vi "Read Anything.vi"(7 "Type of Anything":variant, 8 "Error In":errorcluster, 9 "Section Name (Name of \"Type of Anything\")":string, 11 "Path (dialog)":path) -> (0 "Error Out":errorcluster, 1 "Found?":bool, 3 "Anything":variant)   [LabVIEW 2020]
doc: "This VI is designed to read data from a file written by <B>Write Anything.vi</B>. If the data type definition has changed since it was written to file, this VI will still read and fill out any elements of the cluster that have the same name. Any elements for which it cannot find a name match in the file will be supplied with their datatype's default value.\n\nFreeware from Moore Good Ideas, www.mooregoodideas.com. Do not remove this line."
uses:
  Koop/KObject Class/KObject.lvclass
  <vilib>/Utility/VariantDataType/VariantType.lvlib
  <vilib>/Utility/Data Type/NI_Data Type.lvlib
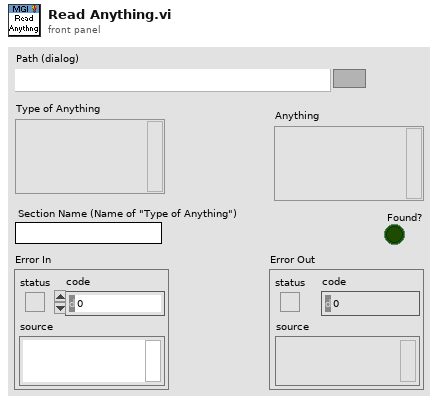
[diagram p1: front panel]
types:
  T1 = typedef "VariantType.lvlib/Type.ctl" = enum8{"Invalid Type", "Void", "I8", "I16", "I32", "I64", "U8", "U16", "U32", "U64", "Single Float", "Double Float", "Extended Float", "Single Complex", "Double Complex", "Extended Complex", "Enum U8", "Enum U16", "Enum U32", "Enum U64", "Single Float With Unit", "Double Float With Unit", "Extended Float With Unit", "Single Complex with Unit", "Double Complex with Unit", "Extended Complex with Unit", "Boolean", "String", "Path", "Picture", "Tag", "Array", "Cluster", "Variant", "LV Variant", "Waveform", "Timestamp", "Digital Waveform", "Digital Data", "ExpressData", "Refnum", "External Data", "VI", "Poly VI", "LabVIEW Class Instance", "Fixed Point"}
  T2 = typedef "NI_Data Type.lvlib/Data Type.ctl" = enum8{"Invalid Type", "Void", "I8", "I16", "I32", "I64", "U8", "U16", "U32", "U64", "Single Float", "Double Float", "Extended Float", "Single Complex", "Double Complex", "Extended Complex", "Enum U8", "Enum U16", "Enum U32", "Enum U64", "Single Float With Unit", "Double Float With Unit", "Extended Float With Unit", "Single Complex with Unit", "Double Complex with Unit", "Extended Complex with Unit", "Boolean", "String", "Path", "Picture", "Tag", "Array", "Cluster", "Variant", "LV Variant", "Waveform", "Timestamp", "Digital Waveform", "Digital Data", "ExpressData", "Refnum", "External Data", "VI", "Poly VI", "LabVIEW Class Instance", "Fixed Point", "Set Collection", "Map Collection"}
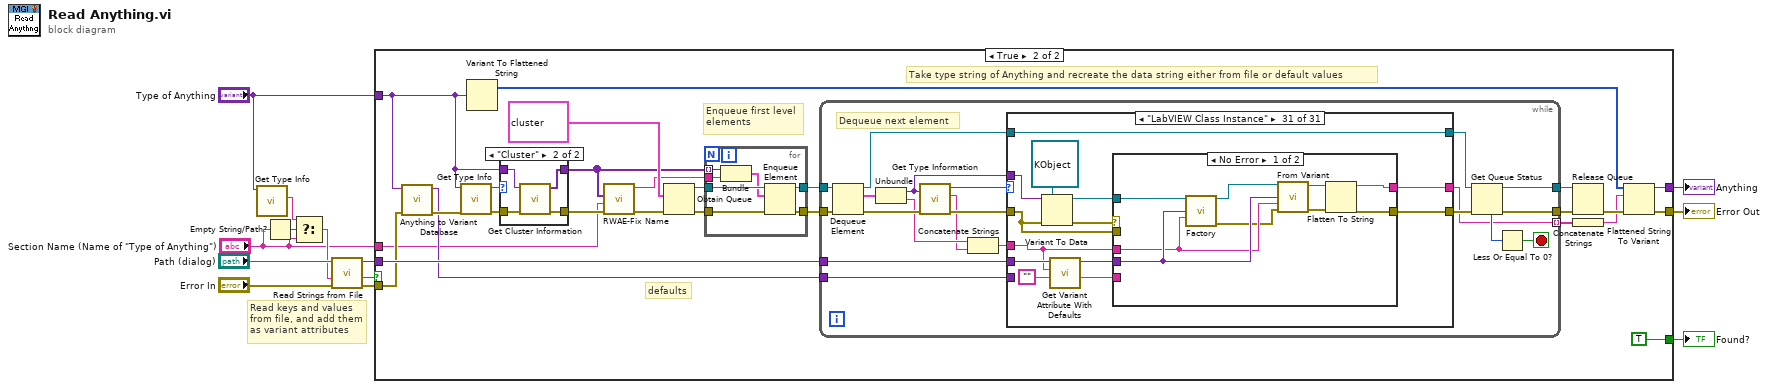
[diagram p0: block diagram]
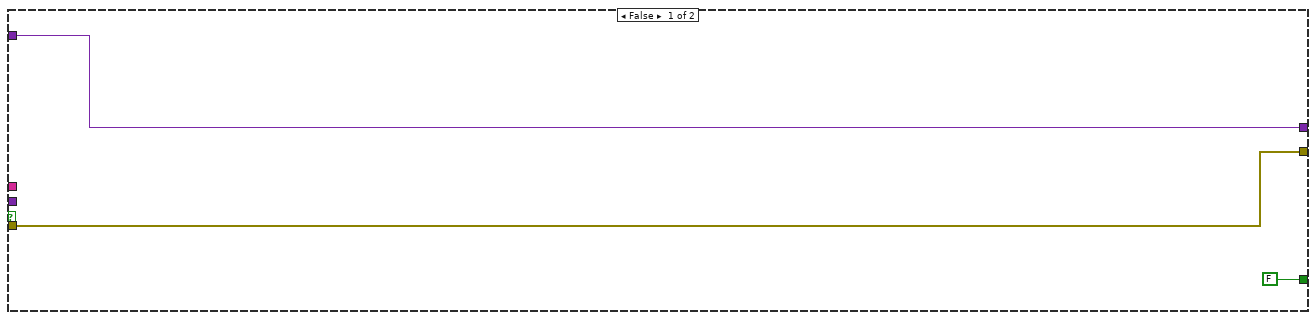
[diagram p2: hidden frame]
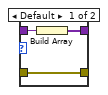
[diagram p3: hidden frame]
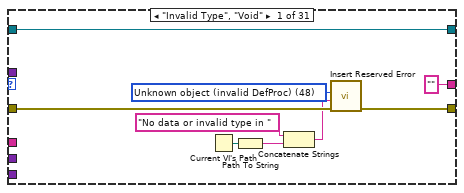
[diagram p4: hidden frame]
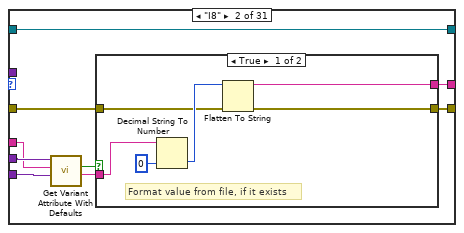
[diagram p5: hidden frame]
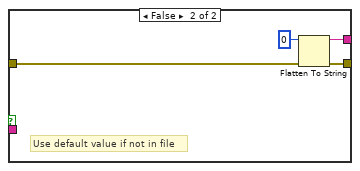
[diagram p6: hidden frame]
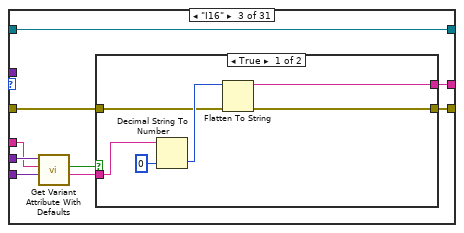
[diagram p7: hidden frame]
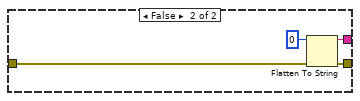
[diagram p8: hidden frame]
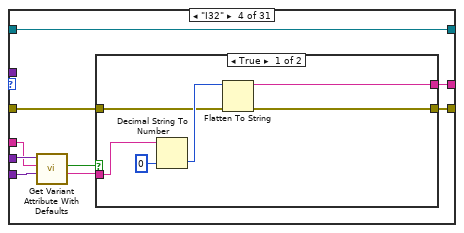
[diagram p9: hidden frame]
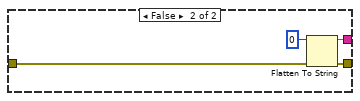
[diagram p10: hidden frame]
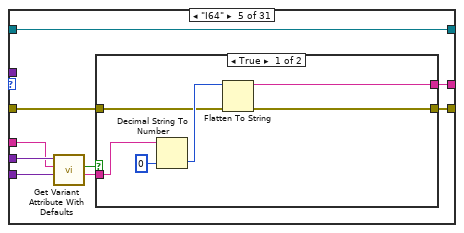
[diagram p11: hidden frame]
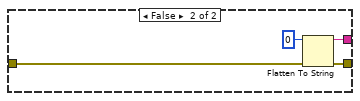
[diagram p12: hidden frame]
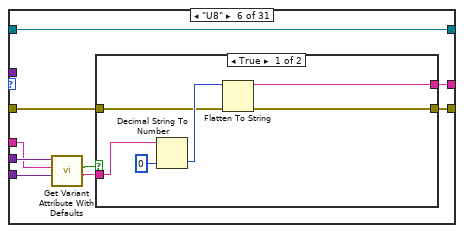
[diagram p13: hidden frame]
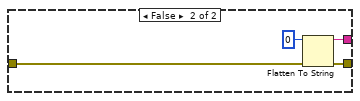
[diagram p14: hidden frame]
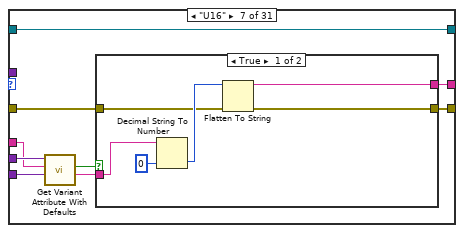
[diagram p15: hidden frame]
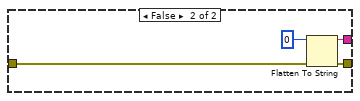
[diagram p16: hidden frame]
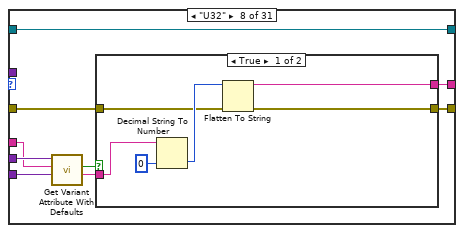
[diagram p17: hidden frame]
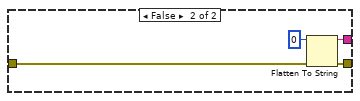
[diagram p18: hidden frame]
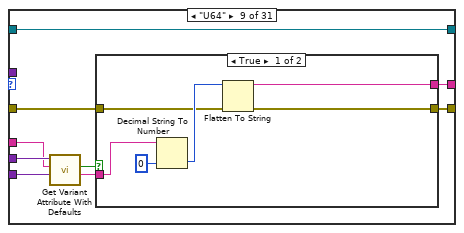
[diagram p19: hidden frame]
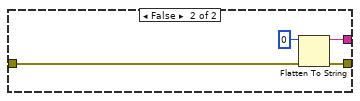
[diagram p20: hidden frame]
diagram:
  # "Read keys and values from file, and add them as variant attributes"
  n1 = call "Get Type Info.vi"("Variant"="Type of Anything") -> ("Name"=w3:string)  [unwired: 8 in, 2 out]
  n2 = Empty String/Path?(string/path="Section Name (Name of \"Type of Anything\")") -> (empty?=w5:bool)
  n3 = Select(t=w3, s=w5, f="Section Name (Name of \"Type of Anything\")") -> (s? t:f=w4:string)
  n4 = call "Read Strings from File.vi"("Error In"="Error In", "Section Name"=w4, "Path"="Path (dialog)") -> ("Error Out"=w11:errorcluster, "Found?"=w8:bool, "Variant Database"=w7:variant)  [unwired: 6 in]
  n5 = case shown="True" w8 {
    tunnel: [w15 w41] -> w13
    tunnel: [w16 w40] -> w12
    tunnel: "Type of Anything" -> [w16 w23]
    tunnel: w11 -> [w15 w25]
    tunnel: [FALSE TRUE] -> w9
    tunnel: w7 -> [_ w28]
    tunnel: "Section Name (Name of \"Type of Anything\")" -> [_ w18]
    frame False {
    }
    frame True {
      # "defaults"
      # "Enqueue first level\nelements"
      # "Take type string of Anything and recreate the data string either from file or default values"
      n6 = call "Anything to Variant Database.vi"("Error In"=w25, "Type of Anything"=w23) -> ("Error Out"=w24:errorcluster, "Variant Database"=w22:variant)  [unwired: 8 in]
      n7 = call "Get Type Info.vi"("Error In"=w24, "Variant"=w23) -> ("Error Out"=w26:errorcluster, "Type Enum"=w27:T1)  [unwired: 7 in, 1 out]
      n8 = Variant To Flattened String(Variant=w23) -> (1:w42:i16[])  [unwired: 1 out]
      n9 = case shown="\"Cluster\"" w27 {
        tunnel: [w45 w48] -> w21
        tunnel: w26 -> [w45 w49]
        tunnel: w23 -> [w44 w47]
        tunnel: [w43 w46] -> w19
        frame Default {
          n10 = Build Array(w44) -> (w43:variant[])
        }
        frame "Cluster" {
          n11 = call <vilib>:"Get Cluster Information.vi"("error in (no error)"=w49, "variant"=w47) -> ("error out"=w48:errorcluster, "cluster elements"=w46:variant[])  [unwired: 8 in]
        }
      }
      n12 = call "RWAE-Fix Name.vi"("error in (no error)"=w21, "Section Name (Name of \"Anything\")"=w18, "Cluster Elements in"=w19) -> ("error out"=w20:errorcluster, "Name"=w17:string)  [unwired: 7 in]
      n13 = Obtain Queue(element data type=cluster{"Variant":variant, "Name":string} {"Variant"=variant, "Name"=""}, error in (no error)=w20) -> (queue out=w38:refnum<queue>, error out=w31:errorcluster)  [unwired: 3 in, 1 out]
      n14 = for {
        tunnel: w38 -> [w56]
        tunnel: [w55] -> w37
        tunnel: [w54] -> w36
        tunnel: w19 -> [w53] mode=indexing
        tunnel: w17 -> [w52]
        tunnel: w31 -> [w51]
        n15 = Bundle("Variant"=w53, "Name"=w52) -> (w50:cluster{"Variant":variant, "Name":string})  [unwired: 1 in]
        n16 = Enqueue Element(queue=w56, element=w50, error in (no error)=w51) -> (queue out=w54:refnum<queue>, error out=w55:errorcluster)  [unwired: 1 in, 1 out]
      }
      n17 = while {
        tunnel: w37 -> [w75]
        tunnel: [w70] -> w35
        tunnel: w28 -> [w62]
        tunnel: [w59] -> w39 mode=indexing
        tunnel: w36 -> [w72]
        tunnel: [w66] -> w33
        tunnel: w22 -> [w58]
        stop <- w67 stop-if-true
        # "Dequeue next element"
        n18 = Dequeue Element(queue=w72, error in (no error)=w75) -> (queue out=w73:refnum<queue>, element=w65:cluster{"Variant":variant, "Name":string}, error out=w74:errorcluster)  [unwired: 1 in, 1 out]
        n19 = Unbundle(w65) -> ("Variant"=w61:variant, "Name"=w63:string)
        n20 = call <vilib>:"Get Type Information.vi"("error in (no error)"=w74, "variant"=w61) -> ("error out"=w76:errorcluster, "name"=w60:string, "type"=w57:T2)  [unwired: 5 in, 2 out]
        n21 = Concatenate Strings(w63, w60) -> (w64:string)
        n22 = case shown="\"LabVIEW Class Instance\"" w57 {
          tunnel: [w79 w94 w113 w132 w151 w170 w189 w208 w227 w246 w265 w284 w303 w322 w341 w361 w387 w413 w439 w464 w483 w500 w517 w539 w568 w597 w626 w655 w683 w695 w719] -> w71
          tunnel: w76 -> [w80 w93 w112 w131 w150 w169 w188 w207 w226 w245 w264 w283 w302 w321 w340 w360 w386 w412 w438 w463 w482 w499 w523 w538 w567 w596 w625 w654 w684 w694 w718]
          tunnel: w64 -> [_ w87 w106 w125 w144 w163 w182 w201 w222 w241 w259 w279 w297 w317 w336 w354 w380 w407 w433 w457 w478 w494 w512 w534 w563 w591 w619 w649 w679 w687 w716]
          tunnel: ["" ("data string") w92 w111 w130 w149 w168 w187 w206 w225 w244 w263 w282 w301 w320 w339 w359 w385 w411 w437 w462 w481 w498 "" w537 w566 w595 w624 w653 w681 w693 w720] -> w59
          tunnel: w61 -> [_ _ _ _ _ _ _ _ _ _ _ _ _ _ _ w358 w384 w410 w436 _ _ _ w522 _ _ _ _ _ w682 _ w721]
          tunnel: w73 -> [w81 w91 w110 w129 w148 w167 w186 w205 w224 w243 w262 w281 w300 w319 w338 w357 w383 w409 w435 w461 w480 w497 w518 w536 w565 w594 w623 w652 w686 w692 w728]
          tunnel: [w81 w91 w110 w129 w148 w167 w186 w205 w224 w243 w262 w281 w300 w319 w338 w357 w383 w409 w435 w461 w480 w497 w516 w536 w565 w594 w623 w652 w685 w692 w728] -> w69
          tunnel: w62 -> [_ w88 w107 w126 w145 w164 w183 w202 w223 w242 w260 w280 w298 w318 w337 w356 w381 w408 w434 w458 w479 w495 _ w535 w564 w593 w622 w650 w680 w690 w726]
          tunnel: w58 -> [_ w86 w105 w124 w143 w162 w181 w200 w219 w238 w257 w276 w295 w314 w333 w352 w378 w404 w430 w456 w475 w492 _ w531 w560 w589 w618 w647 w677 _ _]
          frame "Invalid Type", "Void" {
            w77 = u16 48 items=["No error", "Argument error", "Memory is full", "Out of zone", "End of file", "File already open", "Generic file I/O error", "File not found", "File permission error", "Disk is full", "Duplicate path", "Too many files open", "System feature not enabled", "Resource file not found", "Cannot add resource", "Resource not found", "Image not found", "Image memory error", "Pen does not exist", "Config type invalid", "Config token not found", "Config parse error", "Config memory error", "Bad external code format", "Bad external code offset", "External code not present", "Null window", "Destroy window error", "Null menu", "Print aborted", "Bad print record", "Print driver error", "Windows error during printing", "Memory error during printing", "Print dialog error", "Generic print error", "Invalid device refnum", "Device not found", "Device parameter error", "Device unit error", "Cannot open device", "Device call aborted", "Generic error", "Cancelled by user", "Object ID too low", "Object ID too high", "Object not in heap", "Unknown heap", "Unknown object (invalid DefProc)", "Unknown object (DefProc not in table)", "Message out of range", "Invalid (null) method", "Unknown message", "Manager call not supported", "Bad address", "Network operation in progress", "Network operation timed out", "Connection is busy", "Network attribute not supported", "Network error", "Address in use", "System out of memory", "Connection aborted", "Connection refused", "Not connected", "Already connected", "Connection closed", "Initialization error (interapplication manager)", "Bad occurrence", "Wait on unbound occurrence handler", "Occurrence queue overflow", "Datalog type conflict", "Unused", "Unrecognized type (interapplication manager)", "Memory corrupt", "Failed to make temporary DLL", "Old CIN version", "Drag socket not found", "Failed to load drop-object", "Failed to register OLE object", "Failed to release OLE object", "Format specifier type mismatch", "Unknown format specifier", "Too few format specifiers", "Too many format specifiers", "Scan failed", "Newer CIN version", "OLE Convert", "Runtime menu error", "Password tampered", "Unknown error code"] ("Reserved Error Code")
            n23 = Current VI's Path() -> (path=w83:path)
            n24 = Path To String(path=w83) -> (string=w82:string)
            n25 = Concatenate Strings("No data or invalid type in " ("string"), w82) -> (w78:string)
            n26 = call "Insert Reserved Error.vi"("error in (no error)"=w80, "non-standard source (\"\")"=w78, "Reserved Error Code"=w77) -> ("error out"=w79:errorcluster)  [unwired: 4 in]
          }
          frame "I8" {
            n27 = call "Get Variant Attribute With Defaults.vi"("Variant Database defaults"=w86, "name"=w87, "Variant Database from file"=w88) -> ("values"=w89:string, "found"=w90:bool)  [unwired: 6 in, 1 out]
            n28 = case shown="True" w90 {
              tunnel: w89 -> [w95 _]
              tunnel: [w98 w101] -> w94
              tunnel: w93 -> [w97 w102]
              tunnel: [w99 w104] -> w92
              frame True {
                # "Format value from file, if it exists"
                n29 = Decimal String To Number(string=w95, default (0L)=i8 0 ("default (0 I32)")) -> (number=w100:i8)  [unwired: 1 in, 1 out]
                n30 = Flatten To String(anything=w100, error in (no error)=w97) -> (data string=w99:string, error out=w98:errorcluster)  [unwired: 2 in, 1 out]
              }
              frame False {
                # "Use default value if not in file"
                n31 = Flatten To String(anything=i8 0, error in (no error)=w102) -> (data string=w104:string, error out=w101:errorcluster)  [unwired: 2 in, 1 out]
              }
            }
          }
          frame "I16" {
            n32 = call "Get Variant Attribute With Defaults.vi"("Variant Database defaults"=w105, "name"=w106, "Variant Database from file"=w107) -> ("values"=w108:string, "found"=w109:bool)  [unwired: 6 in, 1 out]
            n33 = case shown="True" w109 {
              tunnel: w108 -> [w114 _]
              tunnel: [w117 w120] -> w113
              tunnel: w112 -> [w116 w121]
              tunnel: [w118 w123] -> w111
              frame True {
                n34 = Decimal String To Number(string=w114, default (0L)=i16 0 ("default (0 I32)")) -> (number=w119:i16)  [unwired: 1 in, 1 out]
                n35 = Flatten To String(anything=w119, error in (no error)=w116) -> (data string=w118:string, error out=w117:errorcluster)  [unwired: 2 in, 1 out]
              }
              frame False {
                n36 = Flatten To String(anything=i16 0, error in (no error)=w121) -> (data string=w123:string, error out=w120:errorcluster)  [unwired: 2 in, 1 out]
              }
            }
          }
          frame "I32" {
            n37 = call "Get Variant Attribute With Defaults.vi"("Variant Database defaults"=w124, "name"=w125, "Variant Database from file"=w126) -> ("values"=w127:string, "found"=w128:bool)  [unwired: 6 in, 1 out]
            n38 = case shown="True" w128 {
              tunnel: w127 -> [w133 _]
              tunnel: [w136 w139] -> w132
              tunnel: w131 -> [w135 w140]
              tunnel: [w137 w142] -> w130
              frame True {
                n39 = Decimal String To Number(string=w133, default (0L)=0 ("default (0 I32)")) -> (number=w138:i32)  [unwired: 1 in, 1 out]
                n40 = Flatten To String(anything=w138, error in (no error)=w135) -> (data string=w137:string, error out=w136:errorcluster)  [unwired: 2 in, 1 out]
              }
              frame False {
                n41 = Flatten To String(anything=0, error in (no error)=w140) -> (data string=w142:string, error out=w139:errorcluster)  [unwired: 2 in, 1 out]
              }
            }
          }
          frame "I64" {
            n42 = call "Get Variant Attribute With Defaults.vi"("Variant Database defaults"=w143, "name"=w144, "Variant Database from file"=w145) -> ("values"=w146:string, "found"=w147:bool)  [unwired: 6 in, 1 out]
            n43 = case shown="True" w147 {
              tunnel: w146 -> [w152 _]
              tunnel: [w155 w158] -> w151
              tunnel: w150 -> [w154 w159]
              tunnel: [w156 w161] -> w149
              frame True {
                n44 = Decimal String To Number(string=w152, default (0L)=i64 0 ("default (0 I32)")) -> (number=w157:i64)  [unwired: 1 in, 1 out]
                n45 = Flatten To String(anything=w157, error in (no error)=w154) -> (data string=w156:string, error out=w155:errorcluster)  [unwired: 2 in, 1 out]
              }
              frame False {
                n46 = Flatten To String(anything=i64 0, error in (no error)=w159) -> (data string=w161:string, error out=w158:errorcluster)  [unwired: 2 in, 1 out]
              }
            }
          }
          frame "U8" {
            n47 = call "Get Variant Attribute With Defaults.vi"("Variant Database defaults"=w162, "name"=w163, "Variant Database from file"=w164) -> ("values"=w165:string, "found"=w166:bool)  [unwired: 6 in, 1 out]
            n48 = case shown="True" w166 {
              tunnel: w165 -> [w171 _]
              tunnel: [w174 w177] -> w170
              tunnel: w169 -> [w173 w178]
              tunnel: [w175 w180] -> w168
              frame True {
                n49 = Decimal String To Number(string=w171, default (0L)=u8 0 ("default (0 I32)")) -> (number=w176:u8)  [unwired: 1 in, 1 out]
                n50 = Flatten To String(anything=w176, error in (no error)=w173) -> (data string=w175:string, error out=w174:errorcluster)  [unwired: 2 in, 1 out]
              }
              frame False {
                n51 = Flatten To String(anything=u8 0, error in (no error)=w178) -> (data string=w180:string, error out=w177:errorcluster)  [unwired: 2 in, 1 out]
              }
            }
          }
          frame "U16" {
            n52 = call "Get Variant Attribute With Defaults.vi"("Variant Database defaults"=w181, "name"=w182, "Variant Database from file"=w183) -> ("values"=w184:string, "found"=w185:bool)  [unwired: 6 in, 1 out]
            n53 = case shown="True" w185 {
              tunnel: w184 -> [w190 _]
              tunnel: [w193 w196] -> w189
              tunnel: w188 -> [w192 w197]
              tunnel: [w194 w199] -> w187
              frame True {
                n54 = Decimal String To Number(string=w190, default (0L)=u16 0 ("default (0 I32)")) -> (number=w195:u16)  [unwired: 1 in, 1 out]
                n55 = Flatten To String(anything=w195, error in (no error)=w192) -> (data string=w194:string, error out=w193:errorcluster)  [unwired: 2 in, 1 out]
              }
              frame False {
                n56 = Flatten To String(anything=u16 0, error in (no error)=w197) -> (data string=w199:string, error out=w196:errorcluster)  [unwired: 2 in, 1 out]
              }
            }
          }
          frame "U32" {
            n57 = call "Get Variant Attribute With Defaults.vi"("Variant Database defaults"=w200, "name"=w201, "Variant Database from file"=w202) -> ("values"=w203:string, "found"=w204:bool)  [unwired: 6 in, 1 out]
            n58 = case shown="True" w204 {
              tunnel: w203 -> [w209 _]
              tunnel: [w212 w215] -> w208
              tunnel: w207 -> [w211 w216]
              tunnel: [w213 w218] -> w206
              frame True {
                n59 = Decimal String To Number(string=w209, default (0L)=u32 0 ("default (0 I32)")) -> (number=w214:u32)  [unwired: 1 in, 1 out]
                n60 = Flatten To String(anything=w214, error in (no error)=w211) -> (data string=w213:string, error out=w212:errorcluster)  [unwired: 2 in, 1 out]
              }
              frame False {
                n61 = Flatten To String(anything=u32 0, error in (no error)=w216) -> (data string=w218:string, error out=w215:errorcluster)  [unwired: 2 in, 1 out]
              }
            }
          }
          frame "U64" {
            n62 = call "Get Variant Attribute With Defaults.vi"("Variant Database defaults"=w219, "name"=w222, "Variant Database from file"=w223) -> ("values"=w221:string, "found"=w220:bool)  [unwired: 6 in, 1 out]
            n63 = case shown="True" w220 {
              tunnel: w221 -> [w228 _]
              tunnel: [w231 w234] -> w227
              tunnel: w226 -> [w230 w235]
              tunnel: [w232 w237] -> w225
              frame True {
                n64 = Decimal String To Number(string=w228, default (0L)=u64 0 ("default (0 I32)")) -> (number=w233:u64)  [unwired: 1 in, 1 out]
                n65 = Flatten To String(anything=w233, error in (no error)=w230) -> (data string=w232:string, error out=w231:errorcluster)  [unwired: 2 in, 1 out]
              }
              frame False {
                n66 = Flatten To String(anything=u64 0, error in (no error)=w235) -> (data string=w237:string, error out=w234:errorcluster)  [unwired: 2 in, 1 out]
              }
            }
          }
          frame "Single Float", "Single Float With Unit" {
            n67 = call "Get Variant Attribute With Defaults.vi"("Variant Database defaults"=w238, "name"=w241, "Variant Database from file"=w242) -> ("values"=w240:string, "found"=w239:bool)  [unwired: 6 in, 1 out]
            n68 = case shown="True" w239 {
              tunnel: w240 -> [w247 _]
              tunnel: [w250 w253] -> w246
              tunnel: w245 -> [w249 w254]
              tunnel: [w251 w256] -> w244
              frame True {
                n69 = Fract/Exp String To Number(string=w247, default (0 dbl)=sgl 0.0 ("default (0 I32)")) -> (number=w252:sgl)  [unwired: 2 in, 1 out]
                n70 = Flatten To String(anything=w252, error in (no error)=w249) -> (data string=w251:string, error out=w250:errorcluster)  [unwired: 2 in, 1 out]
              }
              frame False {
                n71 = Flatten To String(anything=sgl 0.0, error in (no error)=w254) -> (data string=w256:string, error out=w253:errorcluster)  [unwired: 2 in, 1 out]
              }
            }
          }
          frame "Double Float", "Double Float With Unit" {
            n72 = call "Get Variant Attribute With Defaults.vi"("Variant Database defaults"=w257, "name"=w259, "Variant Database from file"=w260) -> ("values"=w261:string, "found"=w258:bool)  [unwired: 6 in, 1 out]
            n73 = case shown="True" w258 {
              tunnel: w261 -> [w266 _]
              tunnel: [w269 w272] -> w265
              tunnel: w264 -> [w268 w273]
              tunnel: [w270 w275] -> w263
              frame True {
                n74 = Fract/Exp String To Number(string=w266, default (0 dbl)=0.0 ("default (0 DBL)")) -> (number=w271:dbl)  [unwired: 2 in, 1 out]
                n75 = Flatten To String(anything=w271, error in (no error)=w268) -> (data string=w270:string, error out=w269:errorcluster)  [unwired: 2 in, 1 out]
              }
              frame False {
                n76 = Flatten To String(anything=0.0, error in (no error)=w273) -> (data string=w275:string, error out=w272:errorcluster)  [unwired: 2 in, 1 out]
              }
            }
          }
          frame "Extended Float", "Extended Float With Unit" {
            n77 = call "Get Variant Attribute With Defaults.vi"("Variant Database defaults"=w276, "name"=w279, "Variant Database from file"=w280) -> ("values"=w278:string, "found"=w277:bool)  [unwired: 6 in, 1 out]
            n78 = case shown="True" w277 {
              tunnel: w278 -> [w285 _]
              tunnel: [w288 w291] -> w284
              tunnel: w283 -> [w287 w292]
              tunnel: [w289 w294] -> w282
              frame True {
                n79 = Fract/Exp String To Number(string=w285, default (0 dbl)=ext 0.0 ("default (0 DBL)")) -> (number=w290:ext)  [unwired: 2 in, 1 out]
                n80 = Flatten To String(anything=w290, error in (no error)=w287) -> (data string=w289:string, error out=w288:errorcluster)  [unwired: 2 in, 1 out]
              }
              frame False {
                n81 = Flatten To String(anything=ext 0.0, error in (no error)=w292) -> (data string=w294:string, error out=w291:errorcluster)  [unwired: 2 in, 1 out]
              }
            }
          }
          frame "Single Complex", "Single Complex with Unit" {
            n82 = call "Get Variant Attribute With Defaults.vi"("Variant Database defaults"=w295, "name"=w297, "Variant Database from file"=w298) -> ("values"=w299:string, "found"=w296:bool)  [unwired: 6 in, 1 out]
            n83 = case shown="True" w296 {
              tunnel: w299 -> [w304 _]
              tunnel: [w308 w310] -> w303
              tunnel: w302 -> [w307 w311]
              tunnel: [w309 w313] -> w301
              frame True {
                n84 = Scan From String(input string=w304, default 1=csg 0.0+0.0i ("default (0 DBL)")) -> (output 1=w305:csg)  [unwired: 3 in, 3 out]
                n85 = Flatten To String(anything=w305, error in (no error)=w307) -> (data string=w309:string, error out=w308:errorcluster)  [unwired: 2 in, 1 out]
              }
              frame False {
                n86 = Flatten To String(anything=csg 0.0+0.0i, error in (no error)=w311) -> (data string=w313:string, error out=w310:errorcluster)  [unwired: 2 in, 1 out]
              }
            }
          }
          frame "Double Complex", "Double Complex with Unit" {
            n87 = call "Get Variant Attribute With Defaults.vi"("Variant Database defaults"=w314, "name"=w317, "Variant Database from file"=w318) -> ("values"=w316:string, "found"=w315:bool)  [unwired: 6 in, 1 out]
            n88 = case shown="True" w315 {
              tunnel: w316 -> [w323 _]
              tunnel: [w327 w329] -> w322
              tunnel: w321 -> [w326 w330]
              tunnel: [w328 w332] -> w320
              frame True {
                n89 = Scan From String(input string=w323, default 1=cdb 0.0+0.0i ("default (0 DBL)")) -> (output 1=w325:cdb)  [unwired: 3 in, 3 out]
                n90 = Flatten To String(anything=w325, error in (no error)=w326) -> (data string=w328:string, error out=w327:errorcluster)  [unwired: 2 in, 1 out]
              }
              frame False {
                n91 = Flatten To String(anything=cdb 0.0+0.0i, error in (no error)=w330) -> (data string=w332:string, error out=w329:errorcluster)  [unwired: 2 in, 1 out]
              }
            }
          }
          frame "Extended Complex", "Extended Complex with Unit" {
            n92 = call "Get Variant Attribute With Defaults.vi"("Variant Database defaults"=w333, "name"=w336, "Variant Database from file"=w337) -> ("values"=w335:string, "found"=w334:bool)  [unwired: 6 in, 1 out]
            n93 = case shown="True" w334 {
              tunnel: w335 -> [w342 _]
              tunnel: [w346 w348] -> w341
              tunnel: w340 -> [w345 w349]
              tunnel: [w347 w351] -> w339
              frame True {
                n94 = Scan From String(input string=w342, default 1=cxt 0.0+0.0i ("default (0 DBL)")) -> (output 1=w343:cxt)  [unwired: 3 in, 3 out]
                n95 = Flatten To String(anything=w343, error in (no error)=w345) -> (data string=w347:string, error out=w346:errorcluster)  [unwired: 2 in, 1 out]
              }
              frame False {
                n96 = Flatten To String(anything=cxt 0.0+0.0i, error in (no error)=w349) -> (data string=w351:string, error out=w348:errorcluster)  [unwired: 2 in, 1 out]
              }
            }
          }
          frame "Enum U8" {
            n97 = call "Get Variant Attribute With Defaults.vi"("Variant Database defaults"=w352, "name"=w354, "Variant Database from file"=w356) -> ("values"=w355:string, "found"=w353:bool)  [unwired: 6 in, 1 out]
            n98 = case shown="True" w353 {
              tunnel: w355 -> [w362 _]
              tunnel: [w372 w375] -> w361
              tunnel: w360 -> [w371 w376]
              tunnel: [w373 w377] -> w359
              tunnel: w358 -> [w370 _]
              frame True {
                n99 = call <vilib>:"GetNumericInfo.vi"("error in (no error)"=w371, "Variant"=w370) -> ("error out"=w363:errorcluster, "EnumNames"=w369:string[])  [unwired: 6 in, 2 out]
                n100 = Search 1D Array(1D array=w369, element=w362) -> (index of element=w368:i32)  [unwired: 1 in]
                n101 = In Range and Coerce(upper limit=255, x=w368, lower limit=0) -> (coerced(x)=w366:i32)  [unwired: 1 out]
                n102 = To Unsigned Byte Integer(number=w366) -> (unsigned 8bit integer=w367:u8)
                n103 = Flatten To String(anything=w367, error in (no error)=w363) -> (data string=w373:string, error out=w372:errorcluster)  [unwired: 2 in, 1 out]
              }
              frame False {
                n104 = Flatten To String(anything=u8 0, error in (no error)=w376) -> (data string=w377:string, error out=w375:errorcluster)  [unwired: 2 in, 1 out]
              }
            }
          }
          frame "Enum U16" {
            n105 = call "Get Variant Attribute With Defaults.vi"("Variant Database defaults"=w378, "name"=w380, "Variant Database from file"=w381) -> ("values"=w382:string, "found"=w379:bool)  [unwired: 6 in, 1 out]
            n106 = case shown="True" w379 {
              tunnel: w382 -> [w388 _]
              tunnel: [w398 w401] -> w387
              tunnel: w386 -> [w397 w402]
              tunnel: [w399 w403] -> w385
              tunnel: w384 -> [w396 _]
              frame True {
                n107 = call <vilib>:"GetNumericInfo.vi"("error in (no error)"=w397, "Variant"=w396) -> ("error out"=w389:errorcluster, "EnumNames"=w395:string[])  [unwired: 6 in, 2 out]
                n108 = Search 1D Array(1D array=w395, element=w388) -> (index of element=w394:i32)  [unwired: 1 in]
                n109 = In Range and Coerce(upper limit=u16 65535, x=w394, lower limit=0) -> (coerced(x)=w392:i32)  [unwired: 1 out]
                n110 = To Unsigned Word Integer(number=w392) -> (unsigned 16bit integer=w393:u16)
                n111 = Flatten To String(anything=w393, error in (no error)=w389) -> (data string=w399:string, error out=w398:errorcluster)  [unwired: 2 in, 1 out]
              }
              frame False {
                n112 = Flatten To String(anything=u16 0, error in (no error)=w402) -> (data string=w403:string, error out=w401:errorcluster)  [unwired: 2 in, 1 out]
              }
            }
          }
          frame "Enum U32" {
            n113 = call "Get Variant Attribute With Defaults.vi"("Variant Database defaults"=w404, "name"=w407, "Variant Database from file"=w408) -> ("values"=w406:string, "found"=w405:bool)  [unwired: 6 in, 1 out]
            n114 = case shown="True" w405 {
              tunnel: w406 -> [w414 _]
              tunnel: [w424 w427] -> w413
              tunnel: w412 -> [w423 w428]
              tunnel: [w425 w429] -> w411
              tunnel: w410 -> [w422 _]
              frame True {
                n115 = call <vilib>:"GetNumericInfo.vi"("error in (no error)"=w423, "Variant"=w422) -> ("error out"=w415:errorcluster, "EnumNames"=w421:string[])  [unwired: 6 in, 2 out]
                n116 = Search 1D Array(1D array=w421, element=w414) -> (index of element=w420:i32)  [unwired: 1 in]
                n117 = In Range and Coerce(upper limit=u32 4294967295, x=w420, lower limit=0) -> (coerced(x)=w418:u32)  [unwired: 1 out]
                n118 = To Unsigned Long Integer(number=w418) -> (unsigned 32bit integer=w419:u32)
                n119 = Flatten To String(anything=w419, error in (no error)=w415) -> (data string=w425:string, error out=w424:errorcluster)  [unwired: 2 in, 1 out]
              }
              frame False {
                n120 = Flatten To String(anything=u32 0, error in (no error)=w428) -> (data string=w429:string, error out=w427:errorcluster)  [unwired: 2 in, 1 out]
              }
            }
          }
          frame "Enum U64" {
            n121 = call "Get Variant Attribute With Defaults.vi"("Variant Database defaults"=w430, "name"=w433, "Variant Database from file"=w434) -> ("values"=w432:string, "found"=w431:bool)  [unwired: 6 in, 1 out]
            n122 = case shown="True" w431 {
              tunnel: [w450 w453] -> w439
              tunnel: w438 -> [w449 w454]
              tunnel: [w451 w455] -> w437
              tunnel: w436 -> [w448 _]
              tunnel: w432 -> [w440 _]
              frame True {
                n123 = call <vilib>:"GetNumericInfo.vi"("error in (no error)"=w449, "Variant"=w448) -> ("error out"=w441:errorcluster, "EnumNames"=w447:string[])  [unwired: 6 in, 2 out]
                n124 = Search 1D Array(1D array=w447, element=w440) -> (index of element=w446:i32)  [unwired: 1 in]
                n125 = In Range and Coerce(upper limit=u64 18446744073709551615, x=w446, lower limit=0) -> (coerced(x)=w444:u64)  [unwired: 1 out]
                n126 = To Unsigned Quad Integer(1:w444) -> (0:w445:u64)
                n127 = Flatten To String(anything=w445, error in (no error)=w441) -> (data string=w451:string, error out=w450:errorcluster)  [unwired: 2 in, 1 out]
              }
              frame False {
                n128 = Flatten To String(anything=u64 0, error in (no error)=w454) -> (data string=w455:string, error out=w453:errorcluster)  [unwired: 2 in, 1 out]
              }
            }
          }
          frame "Boolean" {
            n129 = call "Get Variant Attribute With Defaults.vi"("Variant Database defaults"=w456, "name"=w457, "Variant Database from file"=w458) -> ("values"=w459:string, "found"=w460:bool)  [unwired: 6 in, 1 out]
            n130 = case shown="True" w460 {
              tunnel: w459 -> [w465 _]
              tunnel: [w469 w472] -> w464
              tunnel: w463 -> [w466 w473]
              tunnel: [w470 w474] -> w462
              frame True {
                n131 = Equal?(x=w465, y="TRUE") -> (x = y?=w467:bool)
                n132 = Flatten To String(anything=w467, error in (no error)=w466) -> (data string=w470:string, error out=w469:errorcluster)  [unwired: 2 in, 1 out]
              }
              frame False {
                n133 = Flatten To String(anything=FALSE, error in (no error)=w473) -> (data string=w474:string, error out=w472:errorcluster)  [unwired: 2 in, 1 out]
              }
            }
          }
          frame "String" {
            n134 = call "Get Variant Attribute With Defaults.vi"("Variant Database defaults"=w475, "name"=w478, "Variant Database from file"=w479) -> ("values"=w476:string, "found"=w477:bool)  [unwired: 6 in, 1 out]
            n135 = case shown="True" w477 {
              tunnel: [w486 w489] -> w483
              tunnel: w482 -> [w485 w490]
              tunnel: [w487 w491] -> w481
              tunnel: w476 -> [w484 _]
              frame True {
                n136 = Flatten To String(anything=w484, error in (no error)=w485) -> (data string=w487:string, error out=w486:errorcluster)  [unwired: 2 in, 1 out]
              }
              frame False {
                n137 = Flatten To String(anything="", error in (no error)=w490) -> (data string=w491:string, error out=w489:errorcluster)  [unwired: 2 in, 1 out]
              }
            }
          }
          frame "Path" {
            n138 = call "Get Variant Attribute With Defaults.vi"("Variant Database defaults"=w492, "name"=w494, "Variant Database from file"=w495) -> ("values"=w493:string, "found"=w496:bool)  [unwired: 6 in, 1 out]
            n139 = case shown="True" w496 {
              tunnel: [w504 w507] -> w500
              tunnel: w499 -> [w503 w508]
              tunnel: [w505 w509] -> w498
              tunnel: w493 -> [w501 _]
              frame True {
                n140 = String To Path(string=w501) -> (path=w502:path)
                n141 = Flatten To String(anything=w502, error in (no error)=w503) -> (data string=w505:string, error out=w504:errorcluster)  [unwired: 2 in, 1 out]
              }
              frame False {
                n142 = Flatten To String(anything=path "", error in (no error)=w508) -> (data string=w509:string, error out=w507:errorcluster)  [unwired: 2 in, 1 out]
              }
            }
          }
          frame "Cluster" {
            # "Enqueue cluster elements"
            n143 = call <vilib>:"Search and Replace Pattern.vi"("string"=w512, "regular expression (\"\")"="Serialized") -> ("result string"=w511:string)  [unwired: 3 in, 1 out]
            n144 = call <vilib>:"GetClusterInfo.vi"("error in (no error)"=w523, "Variant"=w522) -> ("error out"=w519:errorcluster, "Cluster Elements"=w521:variant[])  [unwired: 8 in]
            n145 = Concatenate Strings(w511, "." ("string")) -> (w513:string)
            n146 = Reverse 1D Array(array=w521) -> (reversed array=w520:variant[])
            n147 = for {
              tunnel: w518 -> [w530]
              tunnel: w519 -> [w529]
              tunnel: [w528] -> w517
              tunnel: [w527] -> w516
              tunnel: w520 -> [w526] mode=indexing
              tunnel: w513 -> [w524]
              n148 = Bundle("ArrayElt"=w526, w524) -> (w525:cluster{"ArrayElt":variant, string})  [unwired: 1 in]
              n149 = Enqueue Element At Opposite End(queue=w530, element=w525, error in (no error)=w529) -> (queue out=w527:refnum<queue>, error out=w528:errorcluster)  [unwired: 1 in, 1 out]
            }
          }
          frame "Variant", "LV Variant" {
            n150 = call "Get Variant Attribute With Defaults.vi"("Variant Database defaults"=w531, "name"=w534, "Variant Database from file"=w535) -> ("values"=w533:string, "found"=w532:bool)  [unwired: 6 in, 1 out]
            n151 = case shown="True" w532 {
              tunnel: w533 -> [w540 _]
              tunnel: [w548 w557] -> w539
              tunnel: w538 -> [w548 w558]
              tunnel: [w546 w559] -> w537
              frame True {
                n152 = String Subset(string=w540, offset (0)=2) -> (substring=w545:string)  [unwired: 1 in]
                n153 = String Length(string=w545) -> (length=w543:i32)
                n154 = Multiply(x=0.5, y=w543) -> (x*y=w542:dbl)
                n155 = for {
                  N: w542 -> [_]
                  tunnel: w545 -> [w552]
                  tunnel: [w554] -> w544 mode=indexing
                  i -> [w551]
                  w550 = 2 ("length (rest)")
                  n156 = Multiply(x=w551, y=w550) -> (x*y=w549:i32)
                  n157 = String Subset(string=w552, offset (0)=w549, length (rest)=w550) -> (substring=w553:string)
                  n158 = Hexadecimal String To Number(string=w553, default (0uL)=u8 0 ("default (0 U32)")) -> (number=w554:u8)  [unwired: 1 in, 1 out]
                }
                n159 = Byte Array To String(unsigned byte array=w544) -> (string=w546:string)
              }
              frame False {
                w556 = variant  # Variant
                n160 = Flatten To String(anything=w556, error in (no error)=w558) -> (data string=w559:string, error out=w557:errorcluster)  [unwired: 2 in, 1 out]
              }
            }
          }
          frame "Waveform" {
            n161 = call "Get Variant Attribute With Defaults.vi"("Variant Database defaults"=w560, "name"=w563, "Variant Database from file"=w564) -> ("values"=w562:string, "found"=w561:bool)  [unwired: 6 in, 1 out]
            n162 = case shown="False" w561 {
              tunnel: w562 -> [w569 _]
              tunnel: [w577 w587] -> w568
              tunnel: w567 -> [w577 w586]
              tunnel: [w575 w588] -> w566
              frame True {
                n163 = String Subset(string=w569, offset (0)=2) -> (substring=w574:string)  [unwired: 1 in]
                n164 = String Length(string=w574) -> (length=w572:i32)
                n165 = Multiply(x=0.5, y=w572) -> (x*y=w571:dbl)
                n166 = for {
                  N: w571 -> [_]
                  tunnel: w574 -> [w581]
                  tunnel: [w583] -> w573 mode=indexing
                  i -> [w580]
                  w579 = 2 ("length (rest)")
                  n167 = Multiply(x=w580, y=w579) -> (x*y=w578:i32)
                  n168 = String Subset(string=w581, offset (0)=w578, length (rest)=w579) -> (substring=w582:string)
                  n169 = Hexadecimal String To Number(string=w582, default (0uL)=u8 0 ("default (0 U32)")) -> (number=w583:u8)  [unwired: 1 in, 1 out]
                }
                n170 = Byte Array To String(unsigned byte array=w573) -> (string=w575:string)
              }
              frame False {
                n171 = Flatten To String(anything=waveform(dbl) {"t0"=timestamp(0 s since 1904-01-01), "dt"=0.0, "Y"=[]} ("Waveform 2"), error in (no error)=w586) -> (data string=w588:string, error out=w587:errorcluster)  [unwired: 2 in, 1 out]
              }
            }
          }
          frame "Timestamp" {
            n172 = call "Get Variant Attribute With Defaults.vi"("Variant Database defaults"=w589, "name"=w591, "Variant Database from file"=w593) -> ("values"=w592:string, "found"=w590:bool)  [unwired: 6 in, 1 out]
            n173 = case shown="False" w590 {
              tunnel: w592 -> [w598 _]
              tunnel: [w606 w616] -> w597
              tunnel: w596 -> [w606 w615]
              tunnel: [w604 w617] -> w595
              frame True {
                n174 = String Subset(string=w598, offset (0)=2) -> (substring=w603:string)  [unwired: 1 in]
                n175 = String Length(string=w603) -> (length=w601:i32)
                n176 = Multiply(x=0.5, y=w601) -> (x*y=w600:dbl)
                n177 = for {
                  N: w600 -> [_]
                  tunnel: w603 -> [w610]
                  tunnel: [w612] -> w602 mode=indexing
                  i -> [w609]
                  w608 = 2 ("length (rest)")
                  n178 = Multiply(x=w609, y=w608) -> (x*y=w607:i32)
                  n179 = String Subset(string=w610, offset (0)=w607, length (rest)=w608) -> (substring=w611:string)
                  n180 = Hexadecimal String To Number(string=w611, default (0uL)=u8 0 ("default (0 U32)")) -> (number=w612:u8)  [unwired: 1 in, 1 out]
                }
                n181 = Byte Array To String(unsigned byte array=w602) -> (string=w604:string)
              }
              frame False {
                n182 = Flatten To String(anything=timestamp(0 s since 1904-01-01), error in (no error)=w615) -> (data string=w617:string, error out=w616:errorcluster)  [unwired: 2 in, 1 out]
              }
            }
          }
          frame "Digital Waveform" {
            n183 = call "Get Variant Attribute With Defaults.vi"("Variant Database defaults"=w618, "name"=w619, "Variant Database from file"=w622) -> ("values"=w621:string, "found"=w620:bool)  [unwired: 6 in, 1 out]
            n184 = case shown="False" w620 {
              tunnel: w621 -> [w627 _]
              tunnel: [w635 w645] -> w626
              tunnel: w625 -> [w635 w644]
              tunnel: [w633 w646] -> w624
              frame True {
                n185 = String Subset(string=w627, offset (0)=2) -> (substring=w632:string)  [unwired: 1 in]
                n186 = String Length(string=w632) -> (length=w630:i32)
                n187 = Multiply(x=0.5, y=w630) -> (x*y=w629:dbl)
                n188 = for {
                  N: w629 -> [_]
                  tunnel: w632 -> [w639]
                  tunnel: [w641] -> w631 mode=indexing
                  i -> [w638]
                  w637 = 2 ("length (rest)")
                  n189 = Multiply(x=w638, y=w637) -> (x*y=w636:i32)
                  n190 = String Subset(string=w639, offset (0)=w636, length (rest)=w637) -> (substring=w640:string)
                  n191 = Hexadecimal String To Number(string=w640, default (0uL)=u8 0 ("default (0 U32)")) -> (number=w641:u8)  [unwired: 1 in, 1 out]
                }
                n192 = Byte Array To String(unsigned byte array=w631) -> (string=w633:string)
              }
              frame False {
                n193 = call <vilib>:"DWDT Empty Digital.vi"() -> ("digital waveform out"=w643:digitalwaveform)  [unwired: 5 in]
                n194 = Flatten To String(anything=w643, error in (no error)=w644) -> (data string=w646:string, error out=w645:errorcluster)  [unwired: 2 in, 1 out]
              }
            }
          }
          frame "Digital Data" {
            n195 = call "Get Variant Attribute With Defaults.vi"("Variant Database defaults"=w647, "name"=w649, "Variant Database from file"=w650) -> ("values"=w651:string, "found"=w648:bool)  [unwired: 6 in, 1 out]
            n196 = case shown="True" w648 {
              tunnel: w651 -> [w656 _]
              tunnel: [w664 w674] -> w655
              tunnel: w654 -> [w664 w673]
              tunnel: [w662 w675] -> w653
              frame True {
                n197 = String Subset(string=w656, offset (0)=2) -> (substring=w661:string)  [unwired: 1 in]
                n198 = String Length(string=w661) -> (length=w659:i32)
                n199 = Multiply(x=0.5, y=w659) -> (x*y=w658:dbl)
                n200 = for {
                  N: w658 -> [_]
                  tunnel: w661 -> [w668]
                  tunnel: [w670] -> w660 mode=indexing
                  i -> [w667]
                  w666 = 2 ("length (rest)")
                  n201 = Multiply(x=w667, y=w666) -> (x*y=w665:i32)
                  n202 = String Subset(string=w668, offset (0)=w665, length (rest)=w666) -> (substring=w669:string)
                  n203 = Hexadecimal String To Number(string=w669, default (0uL)=u8 0 ("default (0 U32)")) -> (number=w670:u8)  [unwired: 1 in, 1 out]
                }
                n204 = Byte Array To String(unsigned byte array=w660) -> (string=w662:string)
              }
              frame False {
                n205 = call <vilib>:"DTbl Empty Digital.vi"() -> ("digital data"=w672:digitaldata)  [unwired: 5 in]
                n206 = Flatten To String(anything=w672, error in (no error)=w673) -> (data string=w675:string, error out=w674:errorcluster)  [unwired: 2 in, 1 out]
              }
            }
          }
          frame "Array" {
            n207 = call "Get Variant Attribute With Defaults.vi"("Variant Database defaults"=w677, "name"=w679, "Variant Database from file"=w680) -> ("values"=w678:string, "Variant out"=w676:variant)  [unwired: 6 in, 1 out]
            n208 = call "Unprocess Array Elements.vi"("Variant Database"=w676, "Value"=w678, "Error In"=w684, "Name In"=w679, "Array Variant"=w682, "Queue In"=w686) -> ("Error Out"=w683:errorcluster, "Data Out"=w681:string, "Queue Out"=w685:refnum<queue>)  [unwired: 3 in]
          }
          frame Default {
            n209 = call "Get Variant Attribute With Defaults.vi"("Variant Database defaults"="", "name"=w687, "Variant Database from file"=w690) -> ("values"=w689:string, "found"=w688:bool)  [unwired: 6 in, 1 out]
            n210 = case shown="True" w688 {
              tunnel: w689 -> [w696 _]
              tunnel: [w704 w713] -> w695
              tunnel: w694 -> [w704 w714]
              tunnel: [w702 w715] -> w693
              frame True {
                n211 = String Subset(string=w696, offset (0)=2) -> (substring=w701:string)  [unwired: 1 in]
                n212 = String Length(string=w701) -> (length=w699:i32)
                n213 = Multiply(x=0.5, y=w699) -> (x*y=w697:dbl)
                n214 = for {
                  N: w697 -> [_]
                  tunnel: w701 -> [w708]
                  tunnel: [w710] -> w700 mode=indexing
                  i -> [w707]
                  w706 = 2 ("length (rest)")
                  n215 = Multiply(x=w707, y=w706) -> (x*y=w705:i32)
                  n216 = String Subset(string=w708, offset (0)=w705, length (rest)=w706) -> (substring=w709:string)
                  n217 = Hexadecimal String To Number(string=w709, default (0uL)=u8 0 ("default (0 U32)")) -> (number=w710:u8)  [unwired: 1 in, 1 out]
                }
                n218 = Byte Array To String(unsigned byte array=w700) -> (string=w702:string)
              }
              frame False {
                n219 = Flatten To String(anything="", error in (no error)=w714) -> (data string=w715:string, error out=w713:errorcluster)  [unwired: 2 in, 1 out]
              }
            }
          }
          frame "LabVIEW Class Instance" {
            n220 = Variant To Data(error in=w718, type=refnum<class "KObject.lvclass"> refnum ("KObject"), Variant=w721) -> (data=w722:refnum<class "KObject.lvclass">, error out=w723:errorcluster)
            n221 = call "Get Variant Attribute With Defaults.vi"("Variant Database defaults"="", "name"=w716, "Variant Database from file"=w726) -> ("values"=w724:string, "Variant out"=w717:variant)  [unwired: 6 in, 1 out]
            n222 = case shown="No Error" w723 {
              tunnel: w724 -> [_ _]
              tunnel: w722 -> [w731 _]
              tunnel: [w735 _] -> w720
              tunnel: [w736 w738] -> w719
              tunnel: w718 -> [_ w738]
              tunnel: w717 -> [w734 _]
              tunnel: w716 -> [w733 _]
              frame No Error {
                n223 = call-dynamic "Factory.vi"("KObject in"=w731, "Variant"=w734, "Prefix"=w733) -> ("KObject out"=w729:refnum<class "KObject.lvclass">, "error out"=w730:errorcluster)  [unwired: 10 in, 1 out]
                n224 = call-dynamic "From Variant.vi"("KObject in"=w729, "Variant"=w734, "Prefix"=w733, "error in (no error)"=w730) -> ("KObject out"=w732:refnum<class "KObject.lvclass">, "error out"=w737:errorcluster)  [unwired: 10 in]
                n225 = Flatten To String(anything=w732, error in (no error)=w737) -> (data string=w735:string, error out=w736:errorcluster)  [unwired: 2 in, 1 out]
              }
              frame Error {
              }
            }
          }
        }
        n226 = Get Queue Status(queue=w69, error in (no error)=w71) -> (queue out=w66:refnum<queue>, error out=w70:errorcluster, # elements in queue=w68:i32)  [unwired: 1 in, 5 out]
        n227 = Less Or Equal To 0?(x=w68) -> (x <= 0?=w67:bool)
      }
      n228 = Release Queue(queue=w33, error in (no error)=w35) -> (error out=w34:errorcluster)  [unwired: 1 in, 2 out]
      n229 = Concatenate Strings(w39) -> (w29:string)
      n230 = Flattened String To Variant(4:w34, 6:w29, 7:w42) -> (0:w41:errorcluster, 3:w40:variant)
    }
  }
  "Error Out" <- w13
  "Anything" <- w12
  "Found?" <- w9
